vi "get Dll Version Number.vi"() -> (3 "function return":dbl)   [LabVIEW 2023, in "SADI_FW3.lvlib"]
doc: "SADI_API double getDllVersionNumber();"
uses:
  SADI_FW3.lvlib
  SADI_FW3.dll
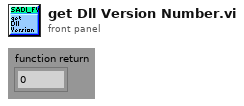
[diagram p1: front panel]
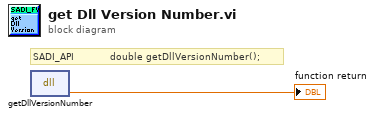
[diagram p0: block diagram]
diagram:
  # "SADI_API            double getDllVersionNumber();"
  n1 = dll-call lib="C:/Users/loran/Documents/School/24_Spring/Controls Lab/EML4314c_Sp24_framework_0/LVLib/SADI_FW3.*" fn="getDllVersionNumber"() -> (→"function return":dbl)  [unwired: 3 in, 2 out]
